vi "Calc Single Distance.vi"(11 "Drive Position Array":dbl[](array[numeric])) -> (3 "mean":dbl)   [LabVIEW 2017, in "WCDrive2018.lvlib"]
uses:
  WCDrive2018.lvlib
  <vilib>/Analysis/baseanly.llb/Mean (DBL).vi
  <vilib>/Analysis/NI_AALBase.lvlib
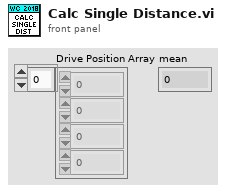
[diagram p1: front panel]
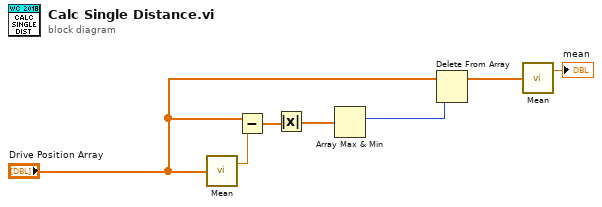
[diagram p0: block diagram]
diagram:
  n1 = call-poly <vilib>:"Mean.vi"("X"="Drive Position Array") -> ("mean"=w1:dbl)  [unwired: 1 out]
  n2 = Subtract(x="Drive Position Array", y=w1) -> (x-y=w2:dbl[])
  n3 = Absolute Value(x=w2) -> (abs(x)=w3:dbl[])
  n4 = Array Max & Min(array=w3) -> (max index (indices)=w5:i32)  [unwired: 3 out]
  n5 = Delete From Array(array="Drive Position Array", index=w5) -> (array with subset deleted=w6:dbl[])  [unwired: 1 in, 1 out]
  n6 = call-poly <vilib>:"Mean.vi"("X"=w6) -> ("mean"=→"mean":dbl)  [unwired: 1 out]
